vi "LKIF_GetCalcData.vi"(8 "error in (no error)":errorcluster {"code" format="%x"}) -> (0 "error out":errorcluster {"code" format="%x"}, 2 "CalcData2":T1 {"LKIF_FLOATRESULT" items=["VALID", "RANGEOVER_P", "RANGEOVER_N", "WAITING"]}, 3 "CalcData1":T1 {"LKIF_FLOATRESULT" items=["VALID", "RANGEOVER_P", "RANGEOVER_N", "WAITING"]})   [LabVIEW 2024, in "Keyence LK-G3000.lvlib"]
uses:
  Keyence LK-G3000.lvlib
  clusters/LKIF_FLOATVALUE.ctl
  enums/LKIF_FLOATRESULT.ctl
panel:
  out "Boolean":bool
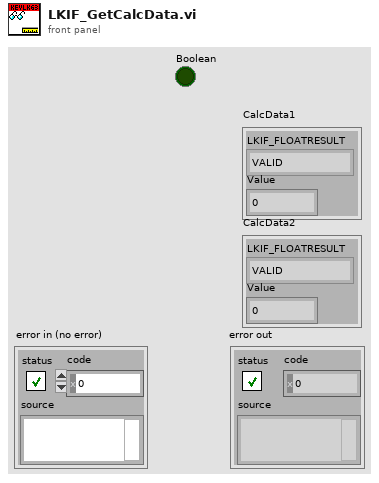
[diagram p1: front panel]
types:
  T1 = typedef "Keyence LK-G3000.lvlib/LKIF_FLOATVALUE.ctl" = cluster{"LKIF_FLOATRESULT":T2, "Value":sgl}
  T2 = typedef "Keyence LK-G3000.lvlib/LKIF_FLOATRESULT.ctl" = i32
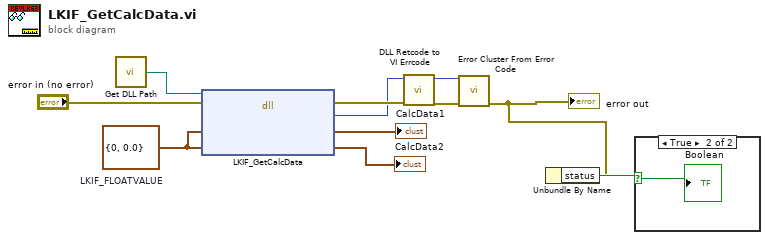
[diagram p0: block diagram]
diagram:
  w6 = T1 {"LKIF_FLOATRESULT"=0, "Value"=0.0}  # LKIF_FLOATVALUE
  n1 = call "Get DLL Path.vi"() -> ("DLL Path"=w7:path)  [unwired: 1 in]
  n2 = dll-call lib="C:/Program Files/National Instruments/LabVIEW 2011/instr.lib/Keyence LK-G3000/LkIF.dll" fn="LKIF_GetCalcData"(path in=w7, error in="error in (no error)", "CalcData1"=w6, "CalcData2"=w6) -> (error out=w9:errorcluster, "RC"=w8:i32, "CalcData1"=→"CalcData1":T1, "CalcData2"=→"CalcData2":T1)  [unwired: 1 in, 1 out]
  n3 = call "DLL Retcode to VI Errcode.vi"("error in (no error)"=w9, "DLL Retcode"=w8) -> ("error out"=w3:errorcluster, "VI Errcode"=w11:i32)  [unwired: 8 in]
  n4 = call <vilib>:"Error Cluster From Error Code.vi"("error in (no error)"=w3, "error code (0)"=w11) -> ("error out"=w1:errorcluster)  [unwired: 7 in]
  "error out" <- w1
  n5 = Unbundle By Name(w1) -> ("status"=w2:bool)
  n6 = case shown="True" w2 {
    selector: w2 -> [_ w12]
    frame False {
    }
    frame True {
      "Boolean" <- w12
    }
  }
